vi "Set Name.vi"(8 "error in":errorcluster, 10 "Name":string, 11 "Class 1 in":refnum<class "Serializer-Scheme.lvclass">) -> (0 "error out":errorcluster, 3 "Class 1 out":refnum<class "Serializer-Scheme.lvclass">)   [LabVIEW 2021, in "TSC Material Theme.lvlib" / "Serializer-Scheme.lvclass"]
uses:
  Serializer-Scheme.lvclass
  Serializer-Scheme.lvclass/Serializer-Scheme.ctl
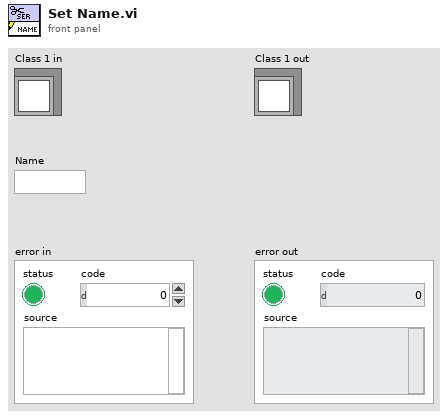
[diagram p1: front panel]
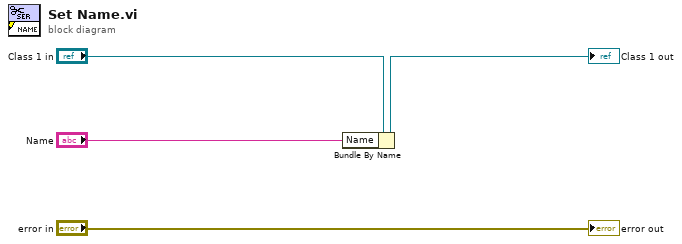
[diagram p0: block diagram]
diagram:
  n1 = Bundle By Name(cluster="Class 1 in", "Name"="Name") -> (→"Class 1 out":refnum<class "Serializer-Scheme.lvclass">)
  "error out" <- "error in"
